vi "IOP Save Data.vi"() -> ()   [LabVIEW 2013]
uses:
  <vilib>/Utility/file.llb/Write To Spreadsheet File (string).vi
  <vilib>/Utility/file.llb/Write To Spreadsheet File (DBL).vi
  Library/KevinLibraryAll/labview/KevLib01.lvlib
panel:
  out "I/A Recording":dbl[](array[numeric])
  out "I/A Pressures":T1(graph)
  out "IOP Recording":dbl[](array[numeric])
  out "Vacuum Cmd":sgl
  out "IOP Pressures":T1(graph)
  out "Threshold Trigger":bool
  out "Vac Chart":sgl(graph)
  out "Elaspsed Time":dbl
  in  "Period [ms]":i64=10
  in  "Seconds of Data":dbl=5.0
  out "File Exists":bool
  in  "Take Data":bool
  in  "File Path":path=path "C:/Users/IRISS/Desktop/IRISSoft/IRISSControl Folder2/Exp Data/data1.txt"
  in  "stop":bool
  # "Pirr\nPvac"
  # "Pac\nPvit"
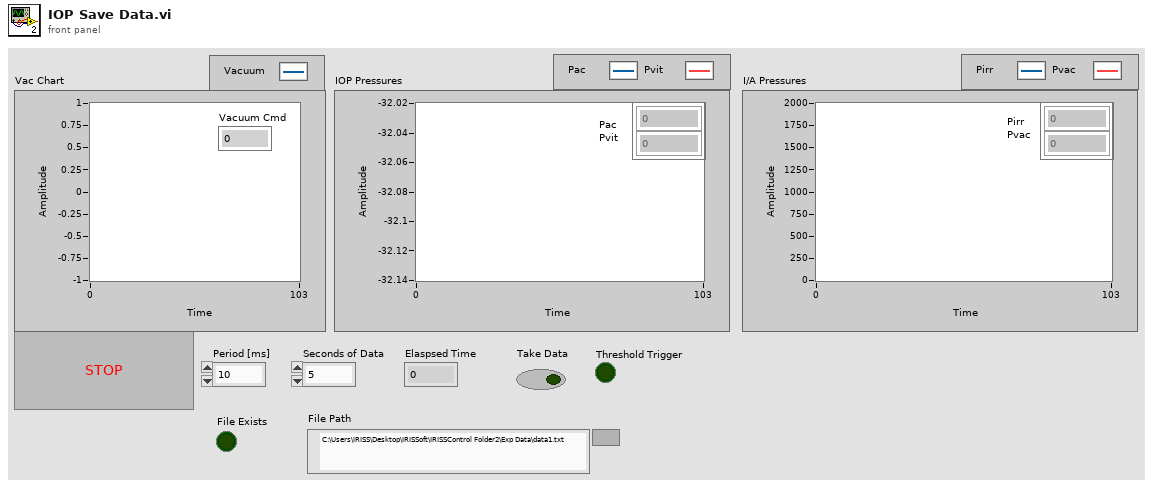
[diagram p1: front panel]
types:
  T1 = cluster{"Array of Double[0]":dbl, "Array of Double[1]":dbl, "Array of Double[2]":dbl, "Array of Double[3]":dbl, "Array of Double[4]":dbl, "Array of Double[5]":dbl, "Array of Double[6]":dbl, "Array of Double[7]":dbl, "Array of Double[8]":dbl}
  T2 = cluster{"[0]":dbl, "[1]":dbl, "[2]":dbl, "[3]":dbl, "[4]":dbl, "[5]":dbl, "[6]":dbl, "[7]":dbl, "[8]":dbl}
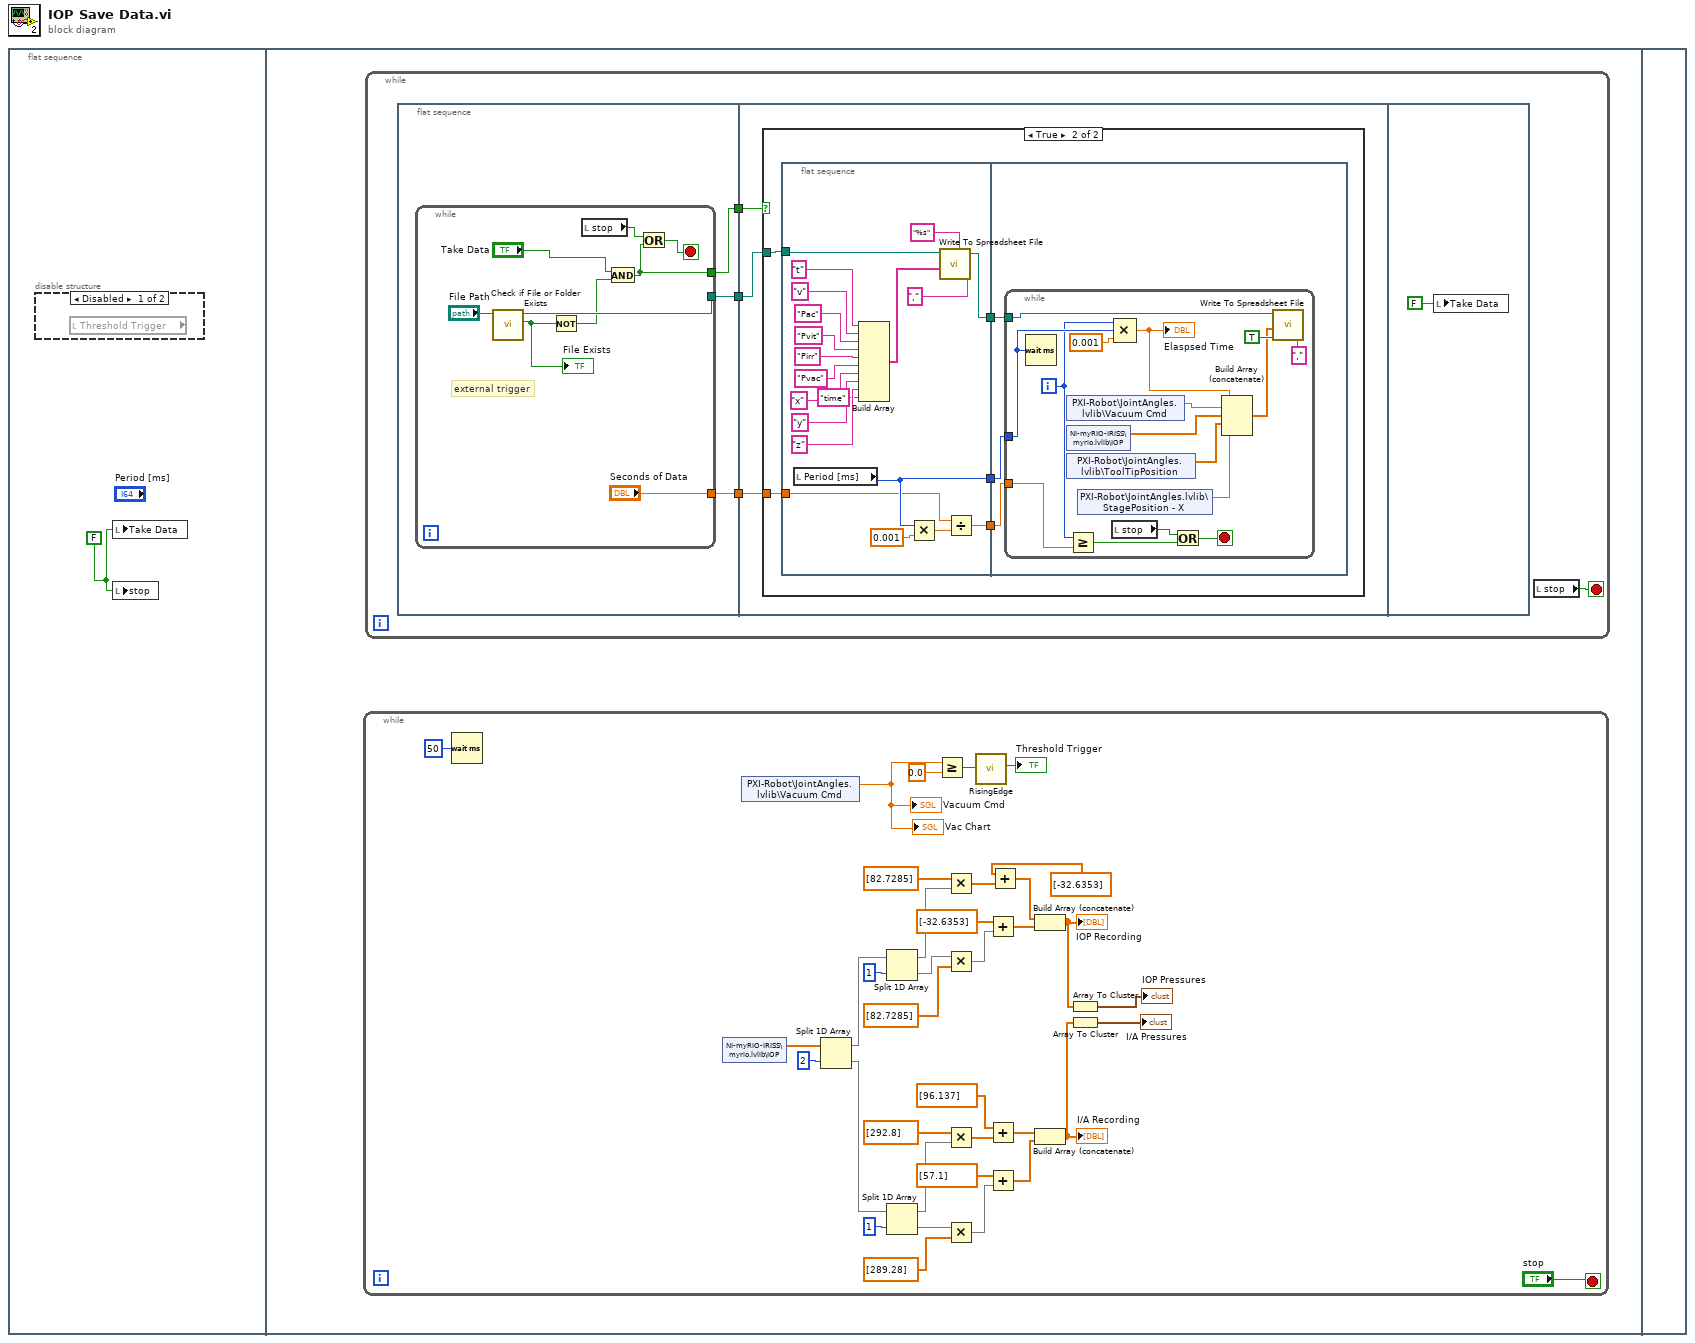
[diagram p0: block diagram]
diagram:
  n1 = flat-sequence {
    frame #0 {
      w1 = FALSE ("stop")
      n2 = disable-structure shown="Disabled" {
        frame Disabled {
          n3 = local read "Threshold Trigger"() -> ()  [unwired: 1 out]
        }
        frame Enabled {
        }
      }
      n4 = local write "Take Data"(w1) -> ()
      n5 = local write "stop"(w1) -> ()
    }
    frame #1 {
      n6 = while {
        stop <- "stop" stop-if-true
        n7 = Wait (ms)(milliseconds to wait=u32 50) -> ()  [unwired: 1 out]
        n8 = shared-variable "NI-myRIO-IRISS\\myrio.lvlib\\IOP"() -> (w6:dbl[])  [unwired: 1 in, 1 out]
        n9 = shared-variable "PXI-Robot\\JointAngles.lvlib\\Vacuum Cmd"() -> (w32:sgl)  [unwired: 1 in, 1 out]
        "Vac Chart" <- w32
        "Vacuum Cmd" <- w32
        n10 = Split 1D Array(array=w6, index=2) -> (first subarray=w30:dbl[], second subarray=w7:dbl[])
        n11 = Split 1D Array(array=w30, index=1) -> (first subarray=w28:dbl[], second subarray=w21:dbl[])
        n12 = Split 1D Array(array=w7, index=1) -> (first subarray=w9:dbl[], second subarray=w16:dbl[])
        n13 = Greater Or Equal?(x=w32, y=sgl 0.0) -> (x >= y?=w34:bool)
        n14 = Multiply(x=dbl[] [82.7285], y=w28) -> (x*y=w26:dbl[])
        n15 = Multiply(x=w21, y=dbl[] [82.7285] ("x")) -> (x*y=w23:dbl[])
        n16 = Multiply(x=dbl[] [292.8], y=w9) -> (x*y=w11:dbl[])
        n17 = Multiply(x=w16, y=dbl[] [289.28] ("x")) -> (x*y=w14:dbl[])
        n18 = call "RisingEdge.vi"("Signal In"=w34) -> ("Rising Edge"=→"Threshold Trigger":bool)  [unwired: 10 in]
        n19 = Add(x=dbl[] [-32.6353], y=w23) -> (x+y=w19:dbl[])
        n20 = Add(x=dbl[] [96.137], y=w11) -> (x+y=w17:dbl[])
        n21 = Add(x=dbl[] [57.1], y=w14) -> (x+y=w18:dbl[])
        n22 = Add(x=dbl[] [-32.6353], y=w26) -> (x+y=w20:dbl[])
        n23 = Build Array (concatenate)(w20, w19) -> (w3:dbl[])
        "IOP Recording" <- w3
        n24 = Build Array (concatenate)(w17, w18) -> (w2:dbl[])
        "I/A Recording" <- w2
        n25 = Array To Cluster(array=w3) -> (cluster=→"IOP Pressures":T2)
        n26 = Array To Cluster(array=w2) -> (cluster=→"I/A Pressures":T2)
      }
      n27 = while {
        stop <- w38 stop-if-true
        n28 = flat-sequence {
          tunnel: [w42] -> w41
          tunnel: [w44] -> w40
          tunnel: [w43] -> w39
          tunnel: w41 -> [w56]
          tunnel: w40 -> [w55]
          tunnel: w39 -> [w54]
          frame #0 {
            n29 = while {
              tunnel: [w51] -> w44
              tunnel: ["Seconds of Data"] -> w43
              tunnel: [w46] -> w42
              stop <- w52 stop-if-true
              # "external trigger"
              n30 = call <vilib>:"Check if File or Folder Exists.vi"("path"="File Path") -> ("file or folder exists?"=w49:bool, "dup path"=w51:path)  [unwired: 8 in, 1 out]
              "File Exists" <- w49
              n31 = Not(x=w49) -> (.not. x?=w48:bool)
              n32 = local read "stop"() -> (w47:bool)
              n33 = And(x="Take Data", y=w48) -> (x .and. y?=w46:bool)
              n34 = Or(x=w47, y=w46) -> (x .or. y?=w52:bool)
            }
          }
          frame #1 {
            n35 = case shown="True" w56 {
              tunnel: w55 -> [_ w61]
              tunnel: w54 -> [_ w58]
              frame False {
              }
              frame True {
                n36 = flat-sequence {
                  tunnel: w61 -> [w75]
                  tunnel: [w74] -> w60
                  tunnel: [w73] -> w59
                  tunnel: w58 -> [w72]
                  tunnel: [w70] -> w57
                  tunnel: w60 -> [w84]
                  tunnel: w59 -> [w83]
                  tunnel: w57 -> [w82]
                  frame #0 {
                    n37 = local read "Period [ms]"() -> (w73:i64)
                    n38 = Build Array("t" ("delimiter (\\t)"), "v" ("delimiter (\\t)"), "Pac" ("delimiter (\\t)"), "Pvit" ("delimiter (\\t)"), "Pirr" ("delimiter (\\t)"), "Pvac" ("delimiter (\\t)"), "x" ("delimiter (\\t)"), "y" ("delimiter (\\t)"), "z" ("delimiter (\\t)"), "time" ("element")) -> (w80:string[])
                    n39 = Multiply(x=w73, y=0.001) -> (x*y=w71:dbl)
                    n40 = call-poly <vilib>:"Write To Spreadsheet File.vi"("delimiter (\\t)"="," ("delimiter (\\t)"), "format (%s)"="%s", "1D data"=w80, "file path (dialog if empty)"=w75) -> ("new file path (Not A Path if cancelled)"=w74:path)  [unwired: 4 in]
                    n41 = Divide(x=w72, y=w71) -> (x/y=w70:dbl)
                  }
                  frame #1 {
                    n42 = while {
                      tunnel: w84 -> [w100]
                      tunnel: w83 -> [w96]
                      tunnel: w82 -> [w94]
                      i -> [w95]
                      stop <- w98 stop-if-true
                      n43 = Wait (ms)(milliseconds to wait=w96) -> ()  [unwired: 1 out]
                      n44 = shared-variable "PXI-Robot\\JointAngles.lvlib\\Vacuum Cmd"() -> (w87:sgl)  [unwired: 1 in, 1 out]
                      n45 = shared-variable "NI-myRIO-IRISS\\myrio.lvlib\\IOP"() -> (w89:dbl[])  [unwired: 1 in, 1 out]
                      n46 = shared-variable "PXI-Robot\\JointAngles.lvlib\\ToolTipPosition"() -> (w86:dbl[])  [unwired: 1 in, 1 out]
                      n47 = Greater Or Equal?(x=w95, y=w94) -> (x >= y?=w93:bool)
                      n48 = shared-variable "PXI-Robot\\JointAngles.lvlib\\StagePosition - X"() -> (w85:dbl)  [unwired: 1 in, 1 out]
                      n49 = local read "stop"() -> (w99:bool)
                      n50 = Compound Arithmetic op=MULTIPLY(w95, w96, 0.001 ("y")) -> (w88:dbl)
                      "Elaspsed Time" <- w88
                      n51 = Or(x=w99, y=w93) -> (x .or. y?=w98:bool)
                      n52 = Build Array (concatenate)(w88, w87, w89, w86, w85) -> (w90:dbl[])
                      n53 = call-poly <vilib>:"Write To Spreadsheet File.vi"("delimiter (\\t)"="," ("delimiter (\\t)"), "append to file? (new file:F)"=TRUE, "1D data"=w90, "file path (dialog if empty)"=w100) -> ()  [unwired: 4 in, 1 out]
                    }
                  }
                }
              }
            }
          }
          frame #2 {
            n54 = local write "Take Data"(FALSE) -> ()
          }
        }
        n55 = local read "stop"() -> (w38:bool)
      }
    }
    frame #2 {
    }
  }
